vi "Write Boolean Configuration.vi"(8 "error in (no error)":errorcluster, 9 "Value":bool, 10 "Name":string, 11 "database-configuration in":refnum<class "configuration-database.lvclass">) -> (0 "error out":errorcluster, 3 "database-configuration out":refnum<class "configuration-database.lvclass">)   [LabVIEW 2020, in "configuration-database.lvlib" / "configuration-database.lvclass"]
uses:
  configuration-database.lvclass
  configuration-database.lvclass/configuration-database.ctl
  22abe498-5327-4947-9dd3-a1594d03bb5b.vi
  <vilib>/Utility/error.llb/Error Cluster From Error Code.vi
  IConfigDBQueries/IConfigurationDatabaseQueries.lvclass
  externals/database-interface/IDatabase/IDatabase/IDatabase.lvclass
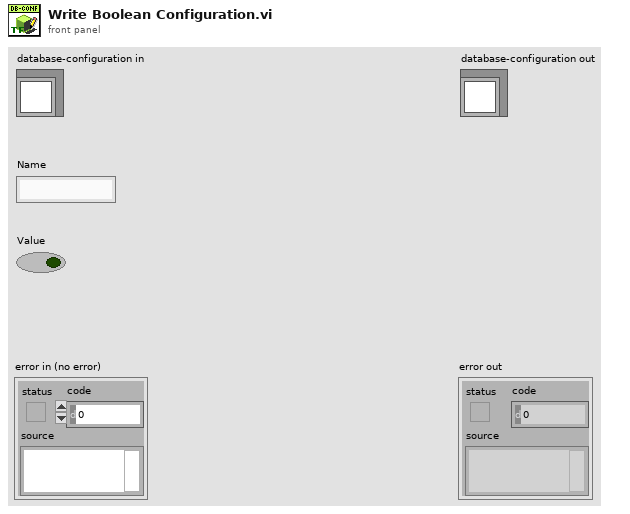
[diagram p1: front panel]
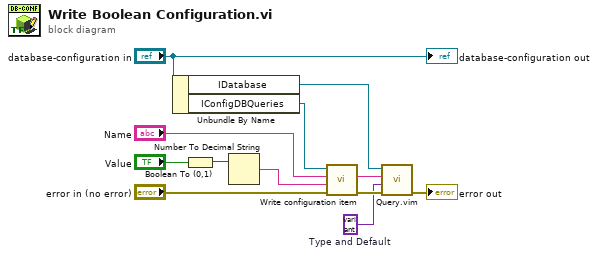
[diagram p0: block diagram]
diagram:
  w1 = variant  # Type and Default
  n1 = Unbundle By Name("database-configuration in") -> ("IDatabase"=w11:refnum<class "IDatabase.lvclass">, "IConfigDBQueries"=w12:refnum<class "IConfigurationDatabaseQueries.lvclass">)
  n2 = Boolean To (0,1)(Boolean="Value") -> (0, 1=w3:i16)
  n3 = Number To Decimal String(number=w3) -> (decimal integer string=w2:string)  [unwired: 1 in]
  n4 = call-dynamic "Write configuration item.vi"("error in (no error)"="error in (no error)", "Value"=w2, "Name in"="Name", "IConfigDBQueries in"=w12) -> ("error out"=w10:errorcluster, "Query"=w9:string)  [unwired: 6 in]
  n5 = call "Query.vim"("error in (no error)"=w10, "Type and Default"=w1, "Query string"=w9, "IDatabase in"=w11) -> ("error out"=→"error out":errorcluster)  [unwired: 5 in, 2 out]
  "database-configuration out" <- "database-configuration in"
